vi "transition.vi"(8 "error in (no error)":errorcluster, 10 "Context In":refnum<class "Context.lvclass">, 11 "Wait Event in":refnum<class "Wait Event.lvclass">) -> (0 "error out":errorcluster, 2 "Context Out":refnum<class "Context.lvclass">, 3 "Wait Event out":refnum<class "Wait Event.lvclass">)   [LabVIEW 2018, in "Wait Event.lvclass"]
uses:
  Wait Event.lvclass
  Context/Context.lvclass
  State/State.lvclass
  ContextData/ContextData.lvclass/ContextData.ctl
  ContextData/ContextData.lvclass
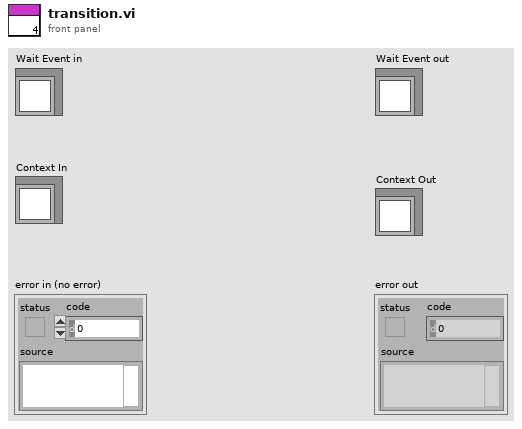
[diagram p1: front panel]
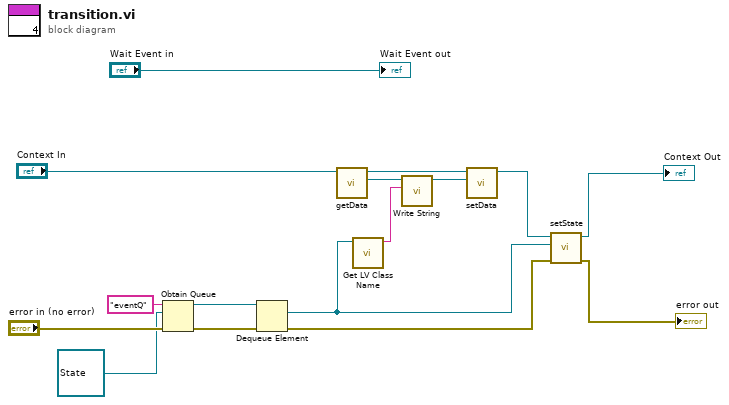
[diagram p0: block diagram]
diagram:
  n1 = Obtain Queue(name (unnamed)="eventQ", element data type=refnum<class "State.lvclass"> refnum ("State.lvclass"), error in (no error)="error in (no error)") -> (queue out=w8:refnum<queue>, error out=w11:errorcluster)  [unwired: 2 in, 1 out]
  n2 = Dequeue Element(queue=w8, error in (no error)=w11) -> (element=w1:refnum<class "State.lvclass">, error out=w12:errorcluster)  [unwired: 1 in, 2 out]
  n3 = call "getData.vi"("Context in"="Context In") -> ("ContextData.lvclass"=w4:refnum<class "ContextData.lvclass">, "Context out"=w6:refnum<class "Context.lvclass">)  [unwired: 8 in, 1 out]
  n4 = call <vilib>:"Get LV Class Name.vi"("object"=w1) -> ("class name"=w2:string)  [unwired: 9 in, 1 out]
  n5 = call "Write String.vi"("String <Replace Me>"=w2, "ContextData in"=w4) -> ("ContextData out"=w3:refnum<class "ContextData.lvclass">)  [unwired: 8 in, 1 out]
  n6 = call "setData.vi"("ContextData.lvclass"=w3, "Context in"=w6) -> ("Context out"=w5:refnum<class "Context.lvclass">)  [unwired: 8 in, 1 out]
  n7 = call "setState.vi"("error in (no error)"=w12, "State.lvclass"=w1, "Context in"=w5) -> ("error out"=→"error out":errorcluster, "Context out"=→"Context Out":refnum<class "Context.lvclass">)  [unwired: 7 in]
  "Wait Event out" <- "Wait Event in"
